vi "check_if_should_flash (SubVI).vi"(6 "Path":path, 7 "Stop below threshold":bool, 8 "Stop threshold":dbl, 9 "Flash lamp?":bool, 10 "Number of cyles\nbetween flashes":i32, 11 "Loop iteration":i32) -> (2 "Curr threshold":dbl, 3 "Should flash":bool)   [LabVIEW 2014]
uses:
  <vilib>/Utility/file.llb/Read From Spreadsheet File (DBL).vi
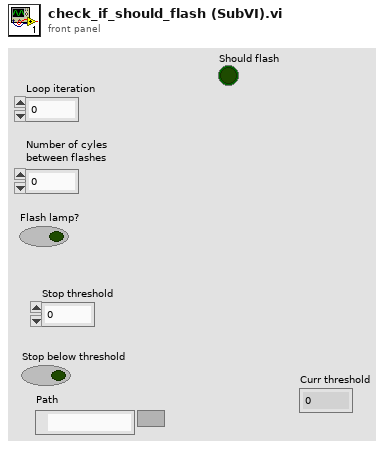
[diagram p1: front panel]
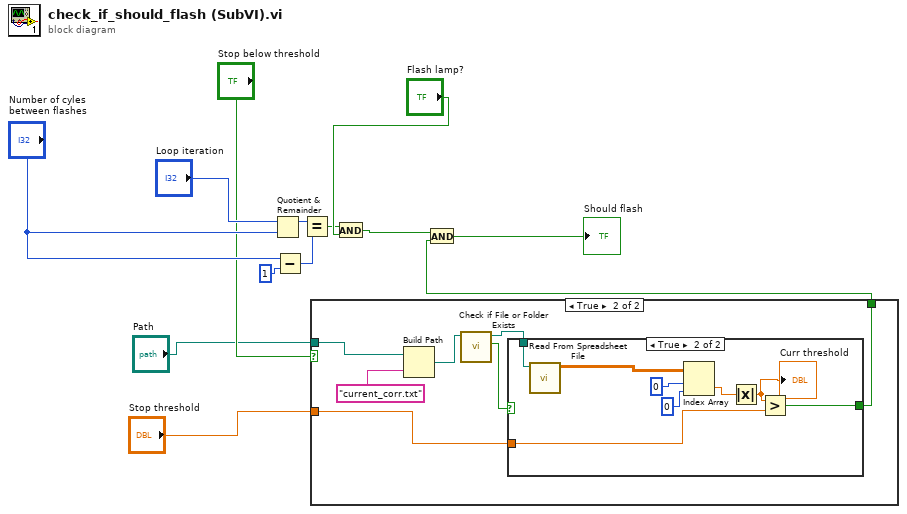
[diagram p0: block diagram]
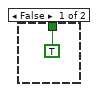
[diagram p2: hidden frame]
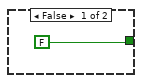
[diagram p3: hidden frame]
diagram:
  n1 = Quotient & Remainder(x="Loop iteration", y="Number of cyles\nbetween flashes") -> (x-y*floor(x/y)=w7:i32)  [unwired: 1 out]
  n2 = Subtract(x="Number of cyles\nbetween flashes", y=1) -> (x-y=w10:i32)
  n3 = Equal?(x=w7, y=w10) -> (x = y?=w11:bool)
  n4 = case shown="True" "Stop below threshold" {
    tunnel: "Path" -> [_ w21]
    tunnel: [TRUE w19] -> w1
    tunnel: "Stop threshold" -> [_ w18]
    frame False {
    }
    frame True {
      n5 = Build Path(base path=w21, name or relative path="current_corr.txt") -> (appended path=w17:path)
      n6 = call <vilib>:"Check if File or Folder Exists.vi"("path"=w17) -> ("file or folder exists?"=w16:bool, "dup path"=w15:path)  [unwired: 8 in, 1 out]
      n7 = case shown="True" w16 {
        tunnel: [FALSE w27] -> w19
        tunnel: w18 -> [_ w24]
        tunnel: w15 -> [_ w23]
        frame False {
        }
        frame True {
          n8 = call-poly <vilib>:"Read From Spreadsheet File.vi"("file path (dialog if empty)"=w23) -> ("all rows"=w30:dbl[][])  [unwired: 6 in, 4 out]
          n9 = Index Array(array=w30, index (row)=0, index (col)=0 ("disabled index (col)")) -> (element=w26:dbl)
          n10 = Absolute Value(x=w26) -> (abs(x)=w25:dbl)
          "Curr threshold" <- w25
          n11 = Greater?(x=w25, y=w24) -> (0:w27:bool)
        }
      }
    }
  }
  n12 = And(x=w11, y="Flash lamp?") -> (x .and. y?=w13:bool)
  n13 = And(x=w13, y=w1) -> (x .and. y?=→"Should flash":bool)
